vi "TS_CustomUI_Init.vi"(0 "TestStand UI ExecutionView Manager":refnum<k7>, 5 "TestStand UI SequenceFileView Manager":refnum<k7>, 7 "TestStand UI Application Manager (in)":refnum<k7>, 9 "VI Refnum":refnum<vi>, 11 "error in":errorcluster, 12 "Controls":T1) -> (4 "TestStand UI Application Manager (out)":refnum<k7>, 6 "Engine Ref out":refnum<k7>, 15 "error out":errorcluster)   [LabVIEW 2010]
uses:
  TS_controls.ctl
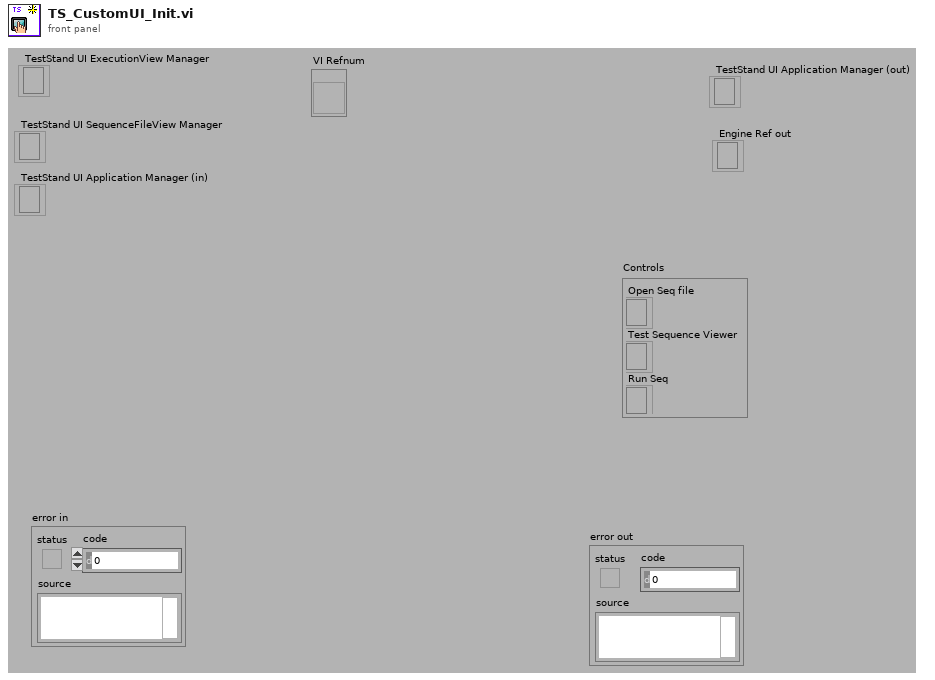
[diagram p1: front panel]
types:
  T1 = typedef "TS_controls.ctl" = cluster{"Open Seq file":refnum<k7>, "Test Sequence Viewer":refnum<k7>, "Run Seq":refnum<k7>}
  T2 = cluster{"TestStand UI ExecutionView Manager":refnum<k7>, "VI Refnum":refnum<vi>, "Test Sequence Viewer":refnum<k7>}
  T3 = cluster{"TestStand UI SequenceFileView Manager":refnum<k7>, "Test Sequence Viewer":refnum<k7>}
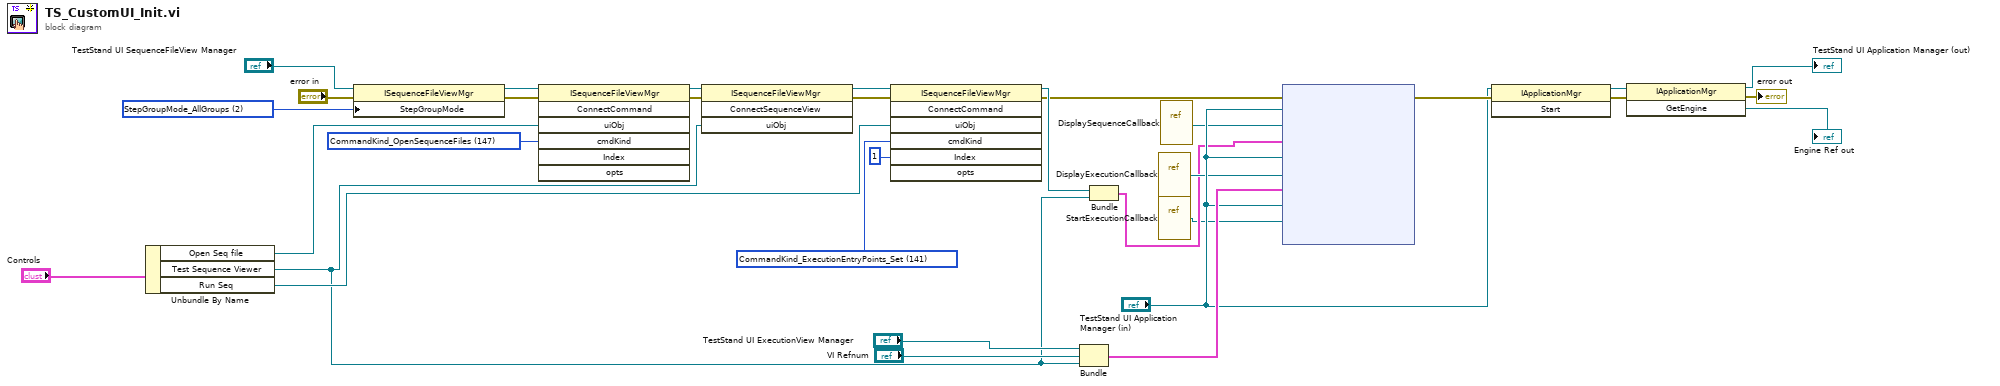
[diagram p0: block diagram]
diagram:
  w19 = 2 items=["StepGroupMode_OneGroup"=1, "StepGroupMode_AllGroups"=2] ("StepGroupMode")
  w27 = 141 items=["CommandKind_NotACommand"=0, "CommandKind_Container"=1, "CommandKind_Separator"=2, "CommandKind_Custom"=3, "CommandKind_OpenSequenceFile"=20, "CommandKind_Close"=21, "CommandKind_CloseAll"=22, "CommandKind_CloseCompletedExecutions"=23, "CommandKind_OpenWorkspaceBrowser"=24, "CommandKind_Login"=25, "CommandKind_Logout"=26, "CommandKind_LoginLogout"=27, "CommandKind_UnloadAllModules"=28, "CommandKind_MRUFile"=29, "CommandKind_Exit"=30, "CommandKind_Restart"=40, "CommandKind_RunEntryPoint"=41, "CommandKind_RunEntryPointOnSelectedSteps"=42, "CommandKind_LoopEntryPointOnSelectedSteps"=43, "CommandKind_RunCurrentSequence"=44, "CommandKind_RunSpecificSequence"=45, "CommandKind_RunSelectedSteps"=46, "CommandKind_RunSelectedStepsUsingEntryPointsSubmenu"=47, "CommandKind_LoopOnSelectedSteps"=48, "CommandKind_LoopOnSelectedStepsUsingEntryPointsSubmenu"=49, "CommandKind_BreakOnFirstStep"=50, "CommandKind_BreakOnStepFailure"=51, "CommandKind_BreakOnSequenceFailure"=52, "CommandKind_TracingEnabled"=53, "CommandKind_ToggleBreakpoint"=60, "CommandKind_SetRunModeSubmenu"=61, "CommandKind_RunModeForcePass"=62, "CommandKind_RunModeForceFail"=63, "CommandKind_RunModeSkip"=64, "CommandKind_RunModeNormal"=65, "CommandKind_Resume"=66, "CommandKind_StepInto"=67, "CommandKind_StepOver"=68, "CommandKind_StepOut"=69, "CommandKind_SetNextStep"=70, "CommandKind_Break"=71, "CommandKind_BreakResume"=72, "CommandKind_Terminate"=73, "CommandKind_TerminateRestart"=74, "CommandKind_Abort"=75, "CommandKind_BreakAll"=76, "CommandKind_TerminateAll"=77, "CommandKind_AbortAll"=78, "CommandKind_ResumeAll"=79, "CommandKind_DisplayBreakpointsAndWatchExpressions"=80, "CommandKind_DisplayBreakpointSettings"=81, "CommandKind_BreakpointSubmenu"=85, "CommandKind_ConfigureAdapters"=90, "CommandKind_ConfigureStationOptions"=91, "CommandKind_ConfigureSearchDirectories"=92, "CommandKind_ConfigureExternalViewers"=93, "CommandKind_ToolItem"=100, "CommandKind_CustomizeTools"=101, "CommandKind_ExecutionEntryPointInsertionMarker"=110, "CommandKind_ExecutionEntryPointDefaultMenuInsertionMarker"=111, "CommandKind_ConfigurationEntryPointInsertionMarker"=112, "CommandKind_ConfigurationEntryPointDefaultMenuInsertionMarker"=113, "CommandKind_SequenceViewConfiguration"=116, "CommandKind_SequenceViewConfigurationsSubmenu"=118, "CommandKind_DefaultFileMenu_Set"=120, "CommandKind_DefaultExecuteMenu_Set"=121, "CommandKind_DefaultDebugMenu_Set"=123, "CommandKind_DefaultConfigureMenu_Set"=124, "CommandKind_DefaultToolsMenu_Set"=125, "CommandKind_DefaultSequenceViewContextMenu_Set"=126, "CommandKind_DefaultListBarContextMenu_Set"=127, "CommandKind_DefaultEditMenu_Set"=128, "CommandKind_DefaultSequenceListContextMenu_Set"=129, "CommandKind_SequenceViewConfigurations_Set"=139, "CommandKind_MRUFiles_Set"=140, "CommandKind_ExecutionEntryPoints_Set"=141, "CommandKind_RunSequences_Set"=142, "CommandKind_RunSelectedStepsUsingEntryPoints_Set"=143, "CommandKind_LoopOnSelectedStepsUsingEntryPoints_Set"=144, "CommandKind_ConfigurationEntryPoints_Set"=145, "CommandKind_Tools_Set"=146, "CommandKind_OpenSequenceFiles"=147, "CommandKind_LockUnlock"=148, "CommandKind_ConfigureSequenceViews"=149, "CommandKind_Edit_Undo"=200, "CommandKind_Edit_Redo"=201, "CommandKind_Edit_Rename"=202, "CommandKind_Edit_Cut"=203, "CommandKind_Edit_Copy"=204, "CommandKind_Edit_Paste"=205, "CommandKind_Edit_Delete"=206, "CommandKind_Edit_InsertStep"=207, "CommandKind_Edit_Save"=208, "CommandKind_Edit_SaveAs"=209, "CommandKind_Edit_SaveAll"=210, "CommandKind_Edit_NewSequenceFile"=211, "CommandKind_Edit_StepProperties"=212, "CommandKind_Edit_SequenceProperties"=213, "CommandKind_Edit_SequenceFileProperties"=214, "CommandKind_Edit_SpecifyModule"=215, "CommandKind_Edit_EditCode"=216, "CommandKind_Edit_EditStep"=217, "CommandKind_Edit_Preconditions"=218, "CommandKind_SelectAll"=219, "CommandKind_Edit_SelectDefaultAdapter"=220, "CommandKind_Edit_InsertSequence"=221, "CommandKind_Edit_SequenceFileCallbacks"=222, "CommandKind_Edit_EditPaths"=223, "CommandKind_Edit_InsertStepsSubmenu"=300, "CommandKind_Edit_EditStepsSubmenu"=301, "CommandKind_Edit_SelectDefaultAdaptersSubmenu"=302, "CommandKind_Edit_InsertSteps_Set"=340, "CommandKind_Edit_EditSteps_Set"=341, "CommandKind_Edit_SelectDefaultAdapters_Set"=342, "CommandKind_ShowInList"=400, "CommandKind_ShowInVariables"=401, "CommandKind_ShowTestStandHelp"=420, "CommandKind_ShowGuideToDocumentation"=421, "CommandKind_ShowHelpTopic"=422, "CommandKind_ShowTestStandWebResources"=423, "CommandKind_ShowTestStandDiscussionForum"=424, "CommandKind_ShowPatents"=425, "CommandKind_DefaultHelpMenu_Set"=440] ("cmdKind")
  w20 = 147 items=["CommandKind_NotACommand"=0, "CommandKind_Container"=1, "CommandKind_Separator"=2, "CommandKind_Custom"=3, "CommandKind_OpenSequenceFile"=20, "CommandKind_Close"=21, "CommandKind_CloseAll"=22, "CommandKind_CloseCompletedExecutions"=23, "CommandKind_OpenWorkspaceBrowser"=24, "CommandKind_Login"=25, "CommandKind_Logout"=26, "CommandKind_LoginLogout"=27, "CommandKind_UnloadAllModules"=28, "CommandKind_MRUFile"=29, "CommandKind_Exit"=30, "CommandKind_Restart"=40, "CommandKind_RunEntryPoint"=41, "CommandKind_RunEntryPointOnSelectedSteps"=42, "CommandKind_LoopEntryPointOnSelectedSteps"=43, "CommandKind_RunCurrentSequence"=44, "CommandKind_RunSpecificSequence"=45, "CommandKind_RunSelectedSteps"=46, "CommandKind_RunSelectedStepsUsingEntryPointsSubmenu"=47, "CommandKind_LoopOnSelectedSteps"=48, "CommandKind_LoopOnSelectedStepsUsingEntryPointsSubmenu"=49, "CommandKind_BreakOnFirstStep"=50, "CommandKind_BreakOnStepFailure"=51, "CommandKind_BreakOnSequenceFailure"=52, "CommandKind_TracingEnabled"=53, "CommandKind_ToggleBreakpoint"=60, "CommandKind_SetRunModeSubmenu"=61, "CommandKind_RunModeForcePass"=62, "CommandKind_RunModeForceFail"=63, "CommandKind_RunModeSkip"=64, "CommandKind_RunModeNormal"=65, "CommandKind_Resume"=66, "CommandKind_StepInto"=67, "CommandKind_StepOver"=68, "CommandKind_StepOut"=69, "CommandKind_SetNextStep"=70, "CommandKind_Break"=71, "CommandKind_BreakResume"=72, "CommandKind_Terminate"=73, "CommandKind_TerminateRestart"=74, "CommandKind_Abort"=75, "CommandKind_BreakAll"=76, "CommandKind_TerminateAll"=77, "CommandKind_AbortAll"=78, "CommandKind_ResumeAll"=79, "CommandKind_DisplayBreakpointsAndWatchExpressions"=80, "CommandKind_DisplayBreakpointSettings"=81, "CommandKind_BreakpointSubmenu"=85, "CommandKind_ConfigureAdapters"=90, "CommandKind_ConfigureStationOptions"=91, "CommandKind_ConfigureSearchDirectories"=92, "CommandKind_ConfigureExternalViewers"=93, "CommandKind_ToolItem"=100, "CommandKind_CustomizeTools"=101, "CommandKind_ExecutionEntryPointInsertionMarker"=110, "CommandKind_ExecutionEntryPointDefaultMenuInsertionMarker"=111, "CommandKind_ConfigurationEntryPointInsertionMarker"=112, "CommandKind_ConfigurationEntryPointDefaultMenuInsertionMarker"=113, "CommandKind_SequenceViewConfiguration"=116, "CommandKind_SequenceViewConfigurationsSubmenu"=118, "CommandKind_DefaultFileMenu_Set"=120, "CommandKind_DefaultExecuteMenu_Set"=121, "CommandKind_DefaultDebugMenu_Set"=123, "CommandKind_DefaultConfigureMenu_Set"=124, "CommandKind_DefaultToolsMenu_Set"=125, "CommandKind_DefaultSequenceViewContextMenu_Set"=126, "CommandKind_DefaultListBarContextMenu_Set"=127, "CommandKind_DefaultEditMenu_Set"=128, "CommandKind_DefaultSequenceListContextMenu_Set"=129, "CommandKind_SequenceViewConfigurations_Set"=139, "CommandKind_MRUFiles_Set"=140, "CommandKind_ExecutionEntryPoints_Set"=141, "CommandKind_RunSequences_Set"=142, "CommandKind_RunSelectedStepsUsingEntryPoints_Set"=143, "CommandKind_LoopOnSelectedStepsUsingEntryPoints_Set"=144, "CommandKind_ConfigurationEntryPoints_Set"=145, "CommandKind_Tools_Set"=146, "CommandKind_OpenSequenceFiles"=147, "CommandKind_LockUnlock"=148, "CommandKind_ConfigureSequenceViews"=149, "CommandKind_Edit_Undo"=200, "CommandKind_Edit_Redo"=201, "CommandKind_Edit_Rename"=202, "CommandKind_Edit_Cut"=203, "CommandKind_Edit_Copy"=204, "CommandKind_Edit_Paste"=205, "CommandKind_Edit_Delete"=206, "CommandKind_Edit_InsertStep"=207, "CommandKind_Edit_Save"=208, "CommandKind_Edit_SaveAs"=209, "CommandKind_Edit_SaveAll"=210, "CommandKind_Edit_NewSequenceFile"=211, "CommandKind_Edit_StepProperties"=212, "CommandKind_Edit_SequenceProperties"=213, "CommandKind_Edit_SequenceFileProperties"=214, "CommandKind_Edit_SpecifyModule"=215, "CommandKind_Edit_EditCode"=216, "CommandKind_Edit_EditStep"=217, "CommandKind_Edit_Preconditions"=218, "CommandKind_SelectAll"=219, "CommandKind_Edit_SelectDefaultAdapter"=220, "CommandKind_Edit_InsertSequence"=221, "CommandKind_Edit_SequenceFileCallbacks"=222, "CommandKind_Edit_EditPaths"=223, "CommandKind_Edit_InsertStepsSubmenu"=300, "CommandKind_Edit_EditStepsSubmenu"=301, "CommandKind_Edit_SelectDefaultAdaptersSubmenu"=302, "CommandKind_Edit_InsertSteps_Set"=340, "CommandKind_Edit_EditSteps_Set"=341, "CommandKind_Edit_SelectDefaultAdapters_Set"=342, "CommandKind_ShowInList"=400, "CommandKind_ShowInVariables"=401, "CommandKind_ShowTestStandHelp"=420, "CommandKind_ShowGuideToDocumentation"=421, "CommandKind_ShowHelpTopic"=422, "CommandKind_ShowTestStandWebResources"=423, "CommandKind_ShowTestStandDiscussionForum"=424, "CommandKind_ShowPatents"=425, "CommandKind_DefaultHelpMenu_Set"=440] ("cmdKind")
  n1 = Unbundle By Name("Controls") -> ("Open Seq file"=w17:refnum<k7>, "Test Sequence Viewer"=w9:refnum<k7>, "Run Seq"=w15:refnum<k7>)
  n2 = property class="ISequenceFileViewMgr"(reference="TestStand UI SequenceFileView Manager", error in="error in", "StepGroupMode"=w19) -> (reference out=w23:refnum<k7>, error out=w32:errorcluster)
  n3 = invoke class="ISequenceFileViewMgr" method="ConnectCommand"(reference=w23, error in=w32, "uiObj"=w17, "cmdKind"=w20) -> (reference out=w22:refnum<k7>, error out=w21:errorcluster)  [unwired: 3 in, 5 out]
  n4 = invoke class="ISequenceFileViewMgr" method="ConnectSequenceView"(reference=w22, error in=w21, "uiObj"=w9) -> (reference out=w25:refnum<k7>, error out=w26:errorcluster)  [unwired: 1 in, 2 out]
  n5 = invoke class="ISequenceFileViewMgr" method="ConnectCommand"(reference=w25, error in=w26, "uiObj"=w15, "cmdKind"=w27, "Index"=1) -> (reference out=w10:refnum<k7>, error out=w7:errorcluster)  [unwired: 2 in, 5 out]
  n6 = Bundle("TestStand UI ExecutionView Manager"="TestStand UI ExecutionView Manager", "VI Refnum"="VI Refnum", "Test Sequence Viewer"=w9) -> (w30:T2)  [unwired: 1 in]
  n7 = Bundle("TestStand UI SequenceFileView Manager"=w10, "Test Sequence Viewer"=w9) -> (w8:T3)  [unwired: 1 in]
  n8 = vi-ref "DisplayExecutionCallback.vi"() -> ("vi reference"=w13:refnum<vi>)
  n9 = vi-ref "StartExecutionCallback.vi"() -> (w1:refnum<vi>)
  n10 = vi-ref "DisplaySequenceCallback.vi"() -> ("vi reference"=w11:refnum<vi>)
  n11 = node(w7, "TestStand UI Application Manager (in)", w11, w8, "TestStand UI Application Manager (in)", w13, w30, "TestStand UI Application Manager (in)", w1) -> (w16:errorcluster)  [unwired: 2 in, 1 out]
  n12 = invoke class="IApplicationMgr" method="Start"(reference="TestStand UI Application Manager (in)", error in=w16) -> (reference out=w6:refnum<k7>, error out=w5:errorcluster)  [unwired: 1 in, 1 out]
  n13 = invoke class="IApplicationMgr" method="GetEngine"(reference=w6, error in=w5) -> (reference out=→"TestStand UI Application Manager (out)":refnum<k7>, error out=→"error out":errorcluster, "GetEngine"=→"Engine Ref out":refnum<k7>)  [unwired: 1 in]
